vi "Keithley 6514 Block Read Setup.vi"(0 "Resource In":refnum<visa-resource-name>, 1 "Check For SCPI Errors? (T)":bool=TRUE, 2 "Time (F)":bool, 3 "Status (F)":bool, 5 "function (Vdc:1)":u16(ring) items=["dc voltage", "resistance", "dc current", "charge"], 7 "Arm Layer Count (1)":i16=1 min=1 max=2500 step=1, 9 "Trigger Layer Count (1)":i16=1 min=1 max=2500 step=1, 11 "error in (no error)":T1, 12 "Trigger Layer Delay (0 secs)":sgl min=0 max=999.9999 step=0.0001 format="%.2f", 13 "Data Type (ASCII:0)":u16(ring) items=["ASCII", "Single Precision REAL"]) -> (4 "Resource Out (dupl)":refnum<visa-resource-name>, 15 "error out":T1)   [LabVIEW 2014, in "KE6514Driver.lvlib"]
doc: "This VI is used prior to executing the 'BLOCK READ' vi with the 6514. The VI allows you to set the function to be measured, the data type , the Arm layer and Trigger layer count values and the trigger delay.\n\nYou may choose to run some of the other VI's that configure the instrument for other parameters such as range, NPLC, or even modify the triggering after this VI has been executed. This VI assumes that the triggering mode will be IMMEDIATE. You may also choose to change the data type or the data elements that are transfered by executing the 'Keithley 6514 Data Format.VI' vi after executing this vi.\n\nGPIB Address:\nDefaults to 14\n\nFunction:\n0 = DC Volts\n1 = Resistance\n2 = DC Current\n3 = Charge\n\nData Type:\n0 = ASCII\n1 = Single Precision Real\n\nArm Layer Count: 1 to 2500\nTrigger Layer Count: 1 to 2500\nNOTE: The result of the arm layer count times the trigger layer count cannot exceed 2500, otherwise an error will result in the 6514.\n\nTrigger Delay: 0 to 999.9999 seconds.\n\nTime:\nFALSE = Off\nTRUE = On\n\nStatus:\nFALSE = Off\nTRUE = On"
uses:
  KE6514Driver.lvlib
panel:
  # "NOTE: The product\nof ARM LAYER COUNT\nand TRIGGER LAYER\nCOUNT cannot exceed 2500"
  # "NOTE: THIS VI MUST BE EXECUTED\nPRIOR TO USING THE 'BLOCK READ' \nVI, OTHERWISE, ERRORS WILL OCCUR."
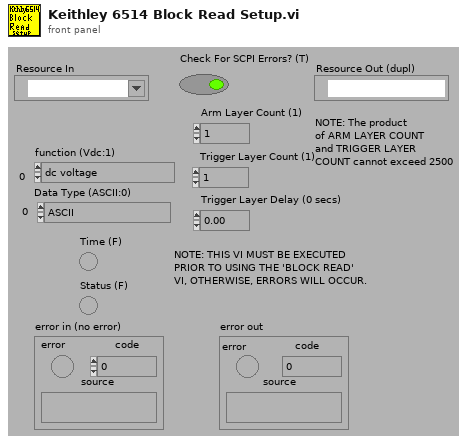
[diagram p1: front panel]
types:
  T1 = cluster{"error":bool, "code":i32, "source":string}
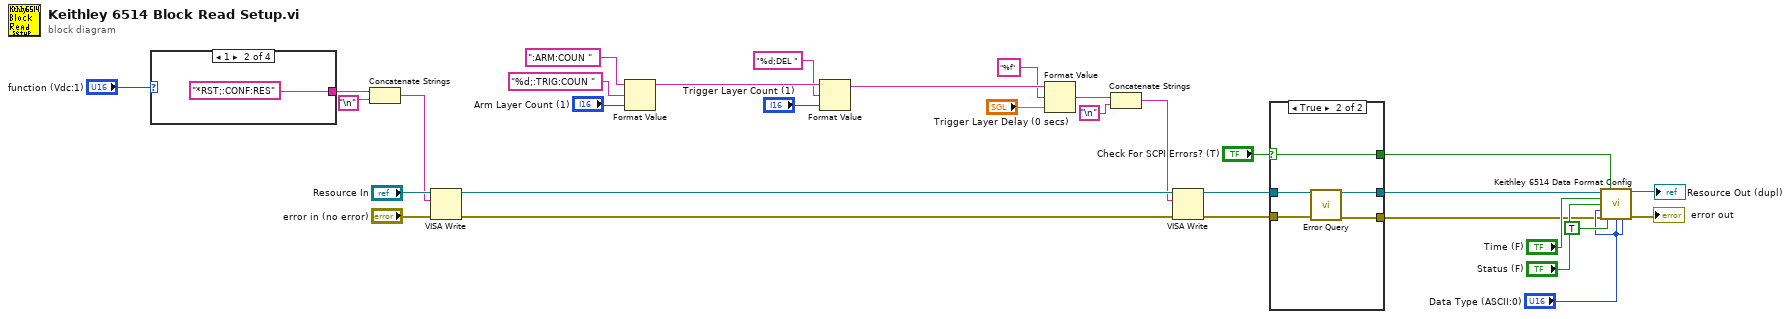
[diagram p0: block diagram]
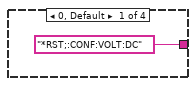
[diagram p3: hidden frame]
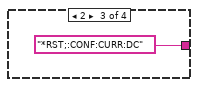
[diagram p4: hidden frame]
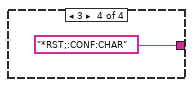
[diagram p5: hidden frame]
diagram:
  n1 = case shown="1" "function (Vdc:1)" {
    tunnel: ["*RST;:CONF:VOLT:DC" "*RST;:CONF:RES" "*RST;:CONF:CURR:DC" "*RST;:CONF:CHAR"] -> w19
    frame 0, Default {
    }
    frame 1 {
    }
    frame 2 {
    }
    frame 3 {
    }
  }
  n2 = Concatenate Strings(w19, "\n") -> (w2:string)
  n3 = VISA Write(VISA resource name="Resource In", write buffer=w2, error in (no error)="error in (no error)") -> (VISA resource name out=w15:refnum<visa-resource-name>, error out=w13:errorcluster)  [unwired: 1 out]
  n4 = Format Value(string ("")=":ARM:COUN ", format string="%d;:TRIG:COUN ", value (0)="Arm Layer Count (1)") -> (output string=w29:string)
  n5 = Format Value(string ("")=w29, format string="%d;DEL ", value (0)="Trigger Layer Count (1)") -> (output string=w28:string)
  n6 = Format Value(string ("")=w28, format string="%f", value (0)="Trigger Layer Delay (0 secs)") -> (output string=w17:string)
  n7 = Concatenate Strings(w17, "\n") -> (w14:string)
  n8 = VISA Write(VISA resource name=w15, write buffer=w14, error in (no error)=w13) -> (VISA resource name out=w8:refnum<visa-resource-name>, error out=w7:errorcluster)  [unwired: 1 out]
  n9 = case shown="True" "Check For SCPI Errors? (T)" {
    selector: "Check For SCPI Errors? (T)" -> [w37 w40]
    tunnel: w8 -> [w39 w44]
    tunnel: w7 -> [w38 w43]
    tunnel: [w39 w42] -> w5
    tunnel: [w38 w41] -> w4
    tunnel: [w37 w40] -> w6
    frame False {
    }
    frame True {
      n10 = call "Error Query.vi"("VISA Resource In"=w44, "error in (no error)"=w43) -> ("VISA Resource Out (dupl)"=w42:refnum<visa-resource-name>, "error out"=w41:errorcluster)  [unwired: 10 in, 2 out]
    }
  }
  n11 = call "Keithley 6514 Data Format Config.vi"("Resource In"=w5, "Check For SCPI Errors? (T)"=w6, "Time (F)"="Time (F)", "Status (F)"="Status (F)", "Data Type (ASCII:0)"="Data Type (ASCII:0)", "error in (no error)"=w4, "Binary Byte Order (Swapped:T))"=TRUE, "Data Format for\nReading Status Registers (ASCII:0)"="Data Type (ASCII:0)", "Data Format for\nReading Output Patterns (ASCII:0)"="Data Type (ASCII:0)") -> ("Resource Out (dupl)"=→"Resource Out (dupl)":refnum<visa-resource-name>, "error out"=→"error out":T1)  [unwired: 5 in]
